vi "UEvent_SET_BYPASS_SHUNT_OR_NOT.vi"(7 "Task in":refnum<k21>, 9 "USB":tag, 10 "Bypass Shunt":T1(ring), 11 "Range_shunt":T2) -> (3 "Task out":refnum<k21>)   [LabVIEW 2015]
uses:
  Range_Shunt_selector.ctl
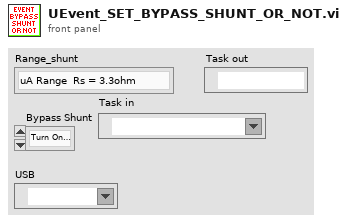
[diagram p1: front panel]
types:
  T1 = enum16{"Turn On bypass - Off Shunt", "Turn Off bypass - On Shunt"}
  T2 = typedef "Range_Shunt_selector.ctl" = enum16{"uA Range  Rs = 3.3ohm", "mA Range Rs = 3.3Ohm", "mA Range Rs = 1Ohm", "mA Range Rs = 1Ohm - X2"}
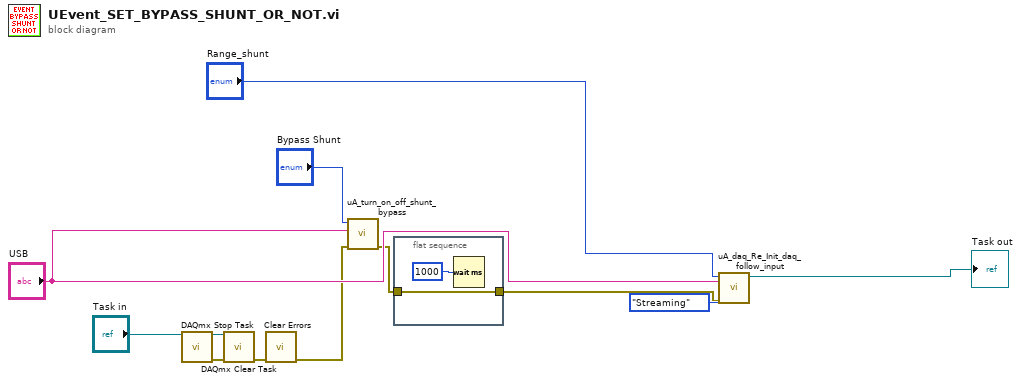
[diagram p0: block diagram]
diagram:
  n1 = call <vilib>:"DAQmx Stop Task.vi"("task/channels in"="Task in") -> ("task out"=w5:refnum<k21>, "error out"=w3:errorcluster)  [unwired: 13 in]
  n2 = call <vilib>:"DAQmx Clear Task.vi"("task in"=w5, "error in"=w3) -> ("error out"=w4:errorcluster)  [unwired: 13 in]
  n3 = call <vilib>:"Clear Errors.vi"("error in (no error)"=w4) -> ("error out"=w1:errorcluster)  [unwired: 5 in, 1 out]
  n4 = call "uA_turn_on_off_shunt_bypass.vi"("error in"=w1, "USB DAQ"="USB", "Bypass Shunt"="Bypass Shunt") -> ("error out"=w9:errorcluster)  [unwired: 8 in]
  n5 = flat-sequence {
    tunnel: w9 -> [w13]
    tunnel: [w13] -> w6
    frame #0 {
      n6 = Wait (ms)(milliseconds to wait=u32 1000) -> ()  [unwired: 1 out]
    }
  }
  n7 = call "uA_daq_Re_Init_daq_follow_input.vi"("error in (no error)"=w6, "Acquire Mode"=enum16{"Streaming", "Read All", "Stop"}."Streaming", "USB"="USB", "Range_shunt"="Range_shunt") -> ("Refnum out"=→"Task out":refnum<k21>)  [unwired: 6 in, 1 out]
